vi "WorkorderHandler_setModifiedData(RemoveLocked).vi"(0 "reference":T1, 2 "data":T2, 5 "error in (no error)":errorcluster) -> (14 "duplicate reference":T1, 19 "error out":errorcluster)   [LabVIEW 2011]
doc: "This VI writes the data of the dqGOOP object and unlocks it for write access. In addition, the locked data is removed from the cache."
uses:
  DataStructures/WorkorderHandler_ObjectReference.ctl
  DataStructures/WorkorderHandler_ObjectData.ctl
panel:
  in  "queue (default)":refnum<queue>
  # "Copyright (C) 2004 DataAct Incorporated"
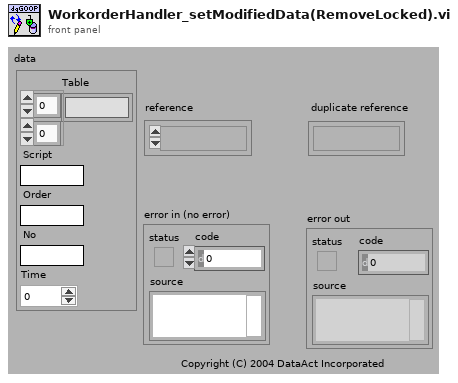
[diagram p1: front panel]
types:
  T1 = typedef "WorkorderHandler_ObjectReference.ctl" = refnum<k1>
  T2 = typedef "WorkorderHandler_ObjectData.ctl" = cluster{"Table":string[][], "Script":string, "Order":string, "No":string, "Time":dbl}
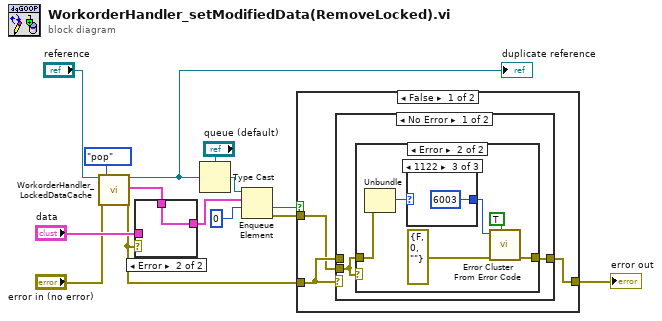
[diagram p0: block diagram]
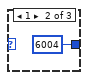
[diagram p5: hidden frame]
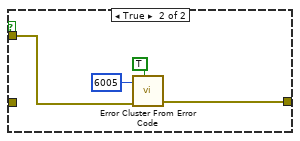
[diagram p7: hidden frame]
diagram:
  n1 = call "WorkorderHandler_LockedDataCache.vi"("reference"="reference", "error in (no error)"="error in (no error)", "action (read)"=enum16{"push", "read", "pop"}."pop" ("action")) -> ("reference dup"=w3:T1, "data out"=w5:T2, "error out"=w1:errorcluster)  [unwired: 1 in, 13 out]
  "duplicate reference" <- w3
  n2 = case shown="Error" w1 {
    tunnel: [w15 w16] -> w11
    tunnel: "data" -> [w15 _]
    tunnel: w5 -> [_ w16]
    frame No Error {
    }
    frame Error {
    }
  }
  n3 = Type Cast(type="queue (default)", x=w3) -> (*(type *) &x=w8:refnum<queue>)
  n4 = Enqueue Element(queue=w8, element=w11, timeout in ms (-1)=0 ("timeout in ms (0)")) -> (timed out?=w13:bool, error out=w7:errorcluster)  [unwired: 1 in, 1 out]
  n5 = case shown="False" w13 {
    tunnel: w1 -> [w19 _]
    tunnel: [w18 w35] -> w14
    tunnel: w7 -> [w17 w33]
    frame False {
      n6 = case shown="No Error" w19 {
        tunnel: [w20 w32] -> w18
        tunnel: w19 -> [_ w32]
        tunnel: w17 -> [w21 _]
        frame No Error {
          n7 = case shown="Error" w21 {
            tunnel: [w22 w23] -> w20
            tunnel: w21 -> [w22 w28]
            frame No Error {
            }
            frame Error {
              n8 = Unbundle(w28) -> ("code"=w27:i32)  [unwired: 2 out]
              n9 = case shown="1122" w27 {
                selector: w27 -> [w29 _ _]
                tunnel: [w29 6004 ("code") 6003 ("code")] -> w25
                frame Default {
                }
                frame 1 {
                }
                frame 1122 {
                }
              }
              n10 = call <vilib>:"Error Cluster From Error Code.vi"("show call chain? (False)"=TRUE, "error in (no error)"=errorcluster {"status"=FALSE, "code"=0, "source"=""} ("error out"), "error code (0)"=w25) -> ("error out"=w23:errorcluster)  [unwired: 6 out]
            }
          }
        }
        frame Error {
        }
      }
    }
    frame True {
      n11 = call <vilib>:"Error Cluster From Error Code.vi"("show call chain? (False)"=TRUE, "error in (no error)"=w33, "error code (0)"=6005 ("code")) -> ("error out"=w35:errorcluster)  [unwired: 6 out]
    }
  }
  "error out" <- w14
